vi "Error Message.vi"(10 "Error Code":i32) -> (2 "Error Message":string)   [LabVIEW 2016, in "Andeen-Hagerling 2700.lvlib"]
doc: "This VI converts a numeric error code from the bridge to an english error message."
uses:
  Andeen-Hagerling 2700.lvlib
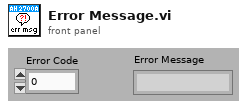
[diagram p1: front panel]
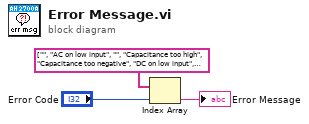
[diagram p0: block diagram]
diagram:
  n1 = Index Array(array=string[] ["", "AC on low input", "", "Capacitance too high", "Capacitance too negative", "DC on low input", "Erratic input", "Excess noise", "", "High to ground short", "High to low short", "Indeterminate off scale", "Low to ground short", "Loss too high", "Loss too negative", "Oven not ready", "Voltage reduced", "Button buffer full", "Ambiguous word", "Bad parameter", "Bad passcode", "Calibration data absent", "Wrong bank", "Calibration data error 0", "Calibration data error 1", "Calibration data error 2", "Calibration data error 3", "Command not operable", "External trigger overrun", "EEPROM error", "File not found", "GPIB output buffer full", "Illegal word", "Internal calibration failure", "Out of space", "Macro nest error", "Syntax error", "Syntax error", "Updated standard error", "Line too long", "", "", "", "", "", "", "", "", "", "", "", "Capacitance deviation too low", "Capacitance deviation too high", "Loss deviation too low", "Loss deviation too high", "Deviation erratic", "Preamp overload", "Deviation conflict", "Units conflict", "Zero conflict", "Deviation initialization failure", "Mode too big", "", "", "", "", "", "", "", "", " ", "", "", "", "", "", "", "Delta conflict", "Floor or ceiling invalid", "No coupled parameter", "Count maximum reached", "", "", "", "No error found", "No data found", "", "", "Deviation span too big", "", "", "Capacitance deviation erratic", "Loss deviation erratic", "Abounds reversal", "Limits reversal", "", "", "", " ", " ", "", "", "", "", "", "", "", "", "", "", " ", "", "", "", "", "", "", "", "", "", "", "", "", "", "", "", "", "", "", "", "", "", "", "", "", "", "", "", " ", " ", "", "", "", "", "", "", "", "", "", "", " ", "", "", "", "", "", "", "", "", "", "", "", "", "", "", "", "", "", "", "", "", "", "", "", "", "", "", "", " ", " ", "", "", "", "", "", "", "", "", "", "", " ", "", "", "", "", "", "", "", "", "", "", "", "", "", "", "", "", "", "", "", "", "", "", "", "", "", "", "", " ", " ", "", "", "", "", "", "", "", "", "", "", " ", "", "", "", "", "", "", "", "", "", "", "", "", "", "", "", "", "", "", ""] ("subarray"), index="Error Code") -> (element=→"Error Message":string)
